vi "Zwangsbedingungen-04-02-17.vi"(4 "AnzahlHorst":i32, 5 "AnzahlHorst/Modul":i32[](array[numeric]), 6 "AnzahlLH":i32, 7 "AnzahlDIOs/Modul":i32[](array[numeric]), 8 "AnzahlDIOs":i32, 9 "Zwangsbedingungen":dbl[][](array[numeric]), 10 "Methodennummer":i32(ring) items=["0"]) -> (1 "Methodennummer":i32(ring) items=["0"])   [LabVIEW 2010]
uses:
  GVMWHorst.vi
  GVHK1Hz.vi
  gvbooleschRT.vi
  GVZeitenZyklen.vi
  GVVentilposition.vi
  GVMetavariablen.vi
  GVZwangs.vi
  GVZwangsMPVPos.vi
  GVZwangsMPV.vi
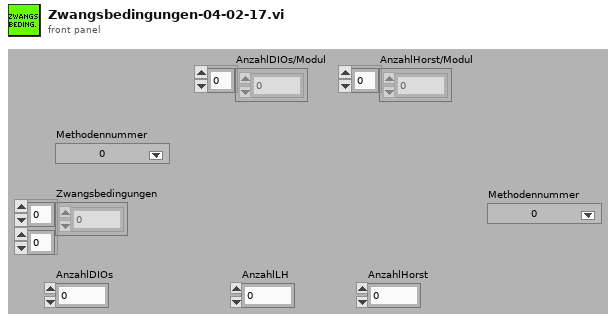
[diagram p1: front panel]
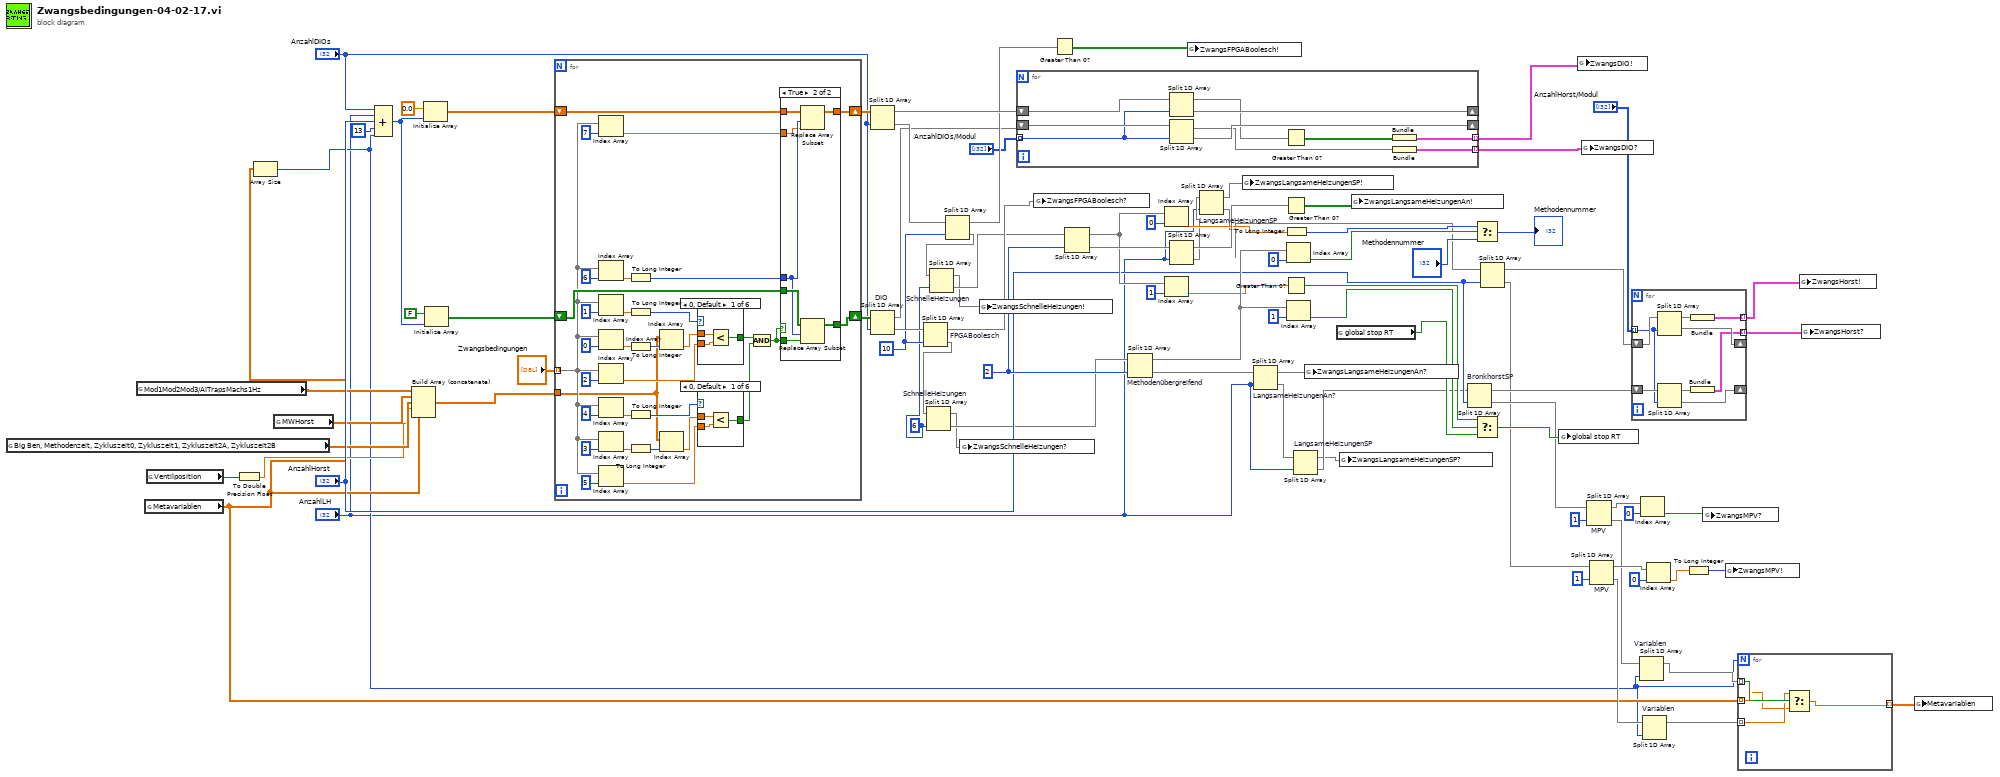
[diagram p0: block diagram]
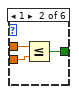
[diagram p2: hidden frame]
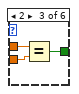
[diagram p3: hidden frame]
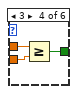
[diagram p4: hidden frame]
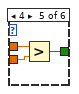
[diagram p5: hidden frame]
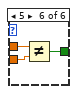
[diagram p6: hidden frame]
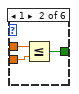
[diagram p8: hidden frame]
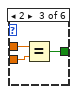
[diagram p9: hidden frame]
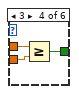
[diagram p10: hidden frame]
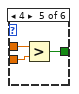
[diagram p11: hidden frame]
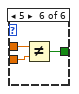
[diagram p12: hidden frame]
diagram:
  w10 = 6 ("index")
  w74 = 2 ("Index")
  w81 = 10 ("Index")
  n1 = global read "GVZeitenZyklen.vi" "Big Ben, Methodenzeit, Zykluszeit0, Zykluszeit1, Zykluszeit2A, Zykluszeit2B"() -> (w35:dbl[])
  n2 = global read "GVHK1Hz.vi" "Mod1Mod2Mod3/AITrapsMachs1Hz"() -> (w38:dbl[])
  n3 = global read "GVMetavariablen.vi" "Metavariablen"() -> (w16:dbl[])
  n4 = global read "GVVentilposition.vi" "Ventilposition"() -> (w34:i32)
  n5 = To Double Precision Float(number=w34) -> (double precision float=w33:dbl)
  n6 = Array Size(array=w16) -> (size(s)=w15:i32)
  n7 = global read "GVMWHorst.vi" "MWHorst"() -> (w47:dbl[])
  n8 = Compound Arithmetic op=ADD("AnzahlDIOs", "AnzahlLH", "AnzahlHorst", 13 ("Wert"), w15) -> (w63:i32)
  n9 = Build Array (concatenate)(w38, w47, w35, w33, w16) -> (w87:dbl[])
  n10 = Initialize Array(0.0, w63) -> (w60:dbl[])
  n11 = Initialize Array(FALSE, w63) -> (w59:bool[])
  n12 = for {
    tunnel: w87 -> [w94]
    tunnel: "Zwangsbedingungen" -> [w98] mode=indexing
    shift-right: [w102] -> w86
    shift-left: w59 -> [w107]
    shift-right: [w103] -> w83
    shift-left: w60 -> [w106]
    n13 = Index Array(array=w98, index=7 ("Index")) -> (element=w104:dbl)
    n14 = Index Array(array=w98, index=6 ("Index")) -> (element=w109:dbl)
    n15 = Index Array(array=w98, index=1 ("Index")) -> (element=w116:dbl)
    n16 = Index Array(array=w98, index=0 ("Index")) -> (element=w118:dbl)
    n17 = Index Array(array=w98, index=2 ("Index")) -> (element=w112:dbl)
    n18 = Index Array(array=w98, index=4 ("Index")) -> (element=w92:dbl)
    n19 = Index Array(array=w98, index=3 ("Index")) -> (element=w93:dbl)
    n20 = Index Array(array=w98, index=5 ("Index")) -> (element=w91:dbl)
    n21 = To Long Integer(number=w109) -> (32bit integer=w105:i32)
    n22 = To Long Integer(number=w116) -> (32bit integer=w115:i32)
    n23 = To Long Integer(number=w118) -> (32bit integer=w111:i32)
    n24 = To Long Integer(number=w92) -> (32bit integer=w97:i32)
    n25 = To Long Integer(number=w93) -> (32bit integer=w95:i32)
    n26 = Index Array(array=w94, index=w111) -> (element=w114:dbl)
    n27 = Index Array(array=w94, index=w95) -> (element=w96:dbl)
    n28 = case shown="0, Default" w115 {
      tunnel: w114 -> [w149 w151 w155 w158 w161 w164]
      tunnel: w112 -> [w148 w152 w154 w157 w160 w163]
      tunnel: [w147 w150 w153 w156 w159 w162] -> w89
      frame 0, Default {
        n29 = Less?(x=w149, y=w148) -> (x < y?=w147:bool)
      }
      frame 1 {
        n30 = Less Or Equal?(x=w151, y=w152) -> (x <= y?=w150:bool)
      }
      frame 2 {
        n31 = Equal?(x=w155, y=w154) -> (x = y?=w153:bool)
      }
      frame 3 {
        n32 = Greater Or Equal?(x=w158, y=w157) -> (x >= y?=w156:bool)
      }
      frame 4 {
        n33 = Greater?(x=w161, y=w160) -> (0:w159:bool)
      }
      frame 5 {
        n34 = Not Equal?(x=w164, y=w163) -> (x != y?=w162:bool)
      }
    }
    n35 = case shown="0, Default" w97 {
      tunnel: w96 -> [w122 w124 w128 w131 w134 w137]
      tunnel: w91 -> [w121 w125 w127 w130 w133 w136]
      tunnel: [w120 w123 w126 w129 w132 w135] -> w90
      frame 0, Default {
        n36 = Less?(x=w122, y=w121) -> (x < y?=w120:bool)
      }
      frame 1 {
        n37 = Less Or Equal?(x=w124, y=w125) -> (x <= y?=w123:bool)
      }
      frame 2 {
        n38 = Equal?(x=w128, y=w127) -> (x = y?=w126:bool)
      }
      frame 3 {
        n39 = Greater Or Equal?(x=w131, y=w130) -> (x >= y?=w129:bool)
      }
      frame 4 {
        n40 = Greater?(x=w134, y=w133) -> (0:w132:bool)
      }
      frame 5 {
        n41 = Not Equal?(x=w137, y=w136) -> (x != y?=w135:bool)
      }
    }
    n42 = And(x=w89, y=w90) -> (x .and. y?=w88:bool)
    n43 = case shown="True" w88 {
      tunnel: w107 -> [w139 w146]
      tunnel: w106 -> [w138 w145]
      tunnel: w105 -> [_ w144]
      tunnel: w88 -> [_ w143]
      tunnel: w104 -> [_ w142]
      tunnel: [w138 w141] -> w103
      tunnel: [w139 w140] -> w102
      frame False {
      }
      frame True {
        n44 = Replace Array Subset(array=w145, new element=w142, index=w144) -> (w141:dbl[])
        n45 = Replace Array Subset(array=w146, new element=w143, index=w144) -> (w140:bool[])
      }
    }
  }
  n46 = Split 1D Array ("DIO")(array=w83, index="AnzahlDIOs") -> (first subarray=w82:dbl[], second subarray=w80:dbl[])
  n47 = Split 1D Array "DIO"(array=w86, index="AnzahlDIOs") -> (first subarray=w69:bool[], second subarray=w85:bool[])
  n48 = Split 1D Array "FPGABoolesch"(array=w85, index=w81) -> (first subarray=w46:bool[], second subarray=w14:bool[])
  n49 = Split 1D Array "SchnelleHeizungen"(array=w14, index=w10) -> (first subarray=w12:bool[], second subarray=w13:bool[])
  n50 = Split 1D Array(array=w80, index=w81) -> (first subarray=w79:dbl[], second subarray=w11:dbl[])
  n51 = Split 1D Array "SchnelleHeizungen"(array=w11, index=w10) -> (first subarray=w8:dbl[], second subarray=w9:dbl[])
  n52 = global write "GVZwangs.vi" "ZwangsSchnelleHeizungen?"(w12) -> ()
  n53 = global write "GVZwangs.vi" "ZwangsSchnelleHeizungen!"(w8) -> ()
  n54 = for {
    tunnel: [w167] -> w41 mode=indexing
    tunnel: "AnzahlDIOs/Modul" -> [w169] mode=indexing
    tunnel: [w165] -> w42 mode=indexing
    shift-right: [w173] -> _
    shift-left: w69 -> [w174]
    shift-right: [w171] -> _
    shift-left: w82 -> [w172]
    n55 = Split 1D Array(array=w172, index=w169) -> (first subarray=w170:dbl[], second subarray=w171:dbl[])
    n56 = Split 1D Array(array=w174, index=w169) -> (first subarray=w168:bool[], second subarray=w173:bool[])
    n57 = Greater Than 0?(x=w170) -> (x > 0?=w166:bool[])
    n58 = Bundle(w166) -> (w165:cluster{bool[]})  [unwired: 1 in]
    n59 = Bundle(w168) -> (w167:cluster{bool[]})  [unwired: 1 in]
  }
  n60 = global write "GVZwangs.vi" "ZwangsFPGABoolesch?"(w46) -> ()
  n61 = Greater Than 0?(x=w79) -> (x > 0?=w45:bool[])
  n62 = Split 1D Array(array=w9, index=w74) -> (first subarray=w70:dbl[], second subarray=w75:dbl[])
  n63 = Split 1D Array "Methodenübergreifend"(array=w13, index=w74) -> (first subarray=w72:bool[], second subarray=w76:bool[])
  n64 = Index Array(array=w70, index=0 ("Index")) -> (element=w52:dbl)
  n65 = Index Array(array=w70, index=1 ("Index")) -> (element=w56:dbl)
  n66 = Split 1D Array(array=w75, index="AnzahlLH") -> (first subarray=w77:dbl[], second subarray=w4:dbl[])
  n67 = global write "GVZwangs.vi" "ZwangsFPGABoolesch!"(w45) -> ()
  n68 = Split 1D Array "LangsameHeizungenSP"(array=w4, index="AnzahlLH") -> (first subarray=w1:dbl[], second subarray=w2:dbl[])
  n69 = global write "GVZwangs.vi" "ZwangsLangsameHeizungenSP!"(w1) -> ()
  n70 = Split 1D Array "LangsameHeizungenAn?"(array=w76, index="AnzahlLH") -> (first subarray=w44:bool[], second subarray=w7:bool[])
  n71 = Greater Than 0?(x=w77) -> (x > 0?=w43:bool[])
  n72 = To Long Integer(number=w52) -> (32bit integer=w50:i32)
  n73 = Greater Than 0?(x=w56) -> (x > 0?=w54:bool)
  n74 = Index Array(array=w72, index=0 ("Index")) -> (element=w51:bool)
  n75 = Index Array(array=w72, index=1 ("Index")) -> (element=w55:bool)
  n76 = Split 1D Array "LangsameHeizungenSP"(array=w7, index="AnzahlLH") -> (first subarray=w5:bool[], second subarray=w6:bool[])
  n77 = global write "GVZwangs.vi" "ZwangsLangsameHeizungenAn?"(w44) -> ()
  n78 = global read "gvbooleschRT.vi" "global stop RT"() -> (w37:bool)
  n79 = global write "GVZwangs.vi" "ZwangsLangsameHeizungenSP?"(w5) -> ()
  n80 = global write "GVZwangs.vi" "ZwangsLangsameHeizungenAn!"(w43) -> ()
  n81 = Split 1D Array "BronkhorstSP"(array=w6, index="AnzahlHorst") -> (first subarray=w84:bool[], second subarray=w32:bool[])
  n82 = Select(t=w50, s=w51, f="Methodennummer") -> (s? t:f=→"Methodennummer":i32)
  n83 = Select(t=w54, s=w55, f=w37) -> (s? t:f=w36:bool)
  n84 = Split 1D Array(array=w2, index="AnzahlHorst") -> (first subarray=w78:dbl[], second subarray=w29:dbl[])
  n85 = global write "gvbooleschRT.vi" "global stop RT"(w36) -> ()
  n86 = global write "GVZwangs.vi" "ZwangsDIO!"(w42) -> ()
  n87 = global write "GVZwangs.vi" "ZwangsDIO?"(w41) -> ()
  n88 = Split 1D Array "MPV"(array=w32, index=1 ("Index")) -> (first subarray=w28:bool[], second subarray=w21:bool[])
  n89 = Split 1D Array "MPV"(array=w29, index=1 ("Index")) -> (first subarray=w24:dbl[], second subarray=w20:dbl[])
  n90 = for {
    tunnel: "AnzahlHorst/Modul" -> [w180] mode=indexing
    shift-right: [w182] -> _
    shift-left: w84 -> [w183]
    tunnel: [w177] -> w39 mode=indexing
    shift-right: [w179] -> _
    shift-left: w78 -> [w181]
    tunnel: [w175] -> w40 mode=indexing
    n91 = Split 1D Array(array=w181, index=w180) -> (first subarray=w176:dbl[], second subarray=w179:dbl[])
    n92 = Split 1D Array(array=w183, index=w180) -> (first subarray=w178:bool[], second subarray=w182:bool[])
    n93 = Bundle(w176) -> (w175:cluster{dbl[]})  [unwired: 1 in]
    n94 = Bundle(w178) -> (w177:cluster{bool[]})  [unwired: 1 in]
  }
  n95 = Split 1D Array "Variablen"(array=w21, index=w15) -> (first subarray=w19:bool[])  [unwired: 1 out]
  n96 = Index Array(array=w28, index=0 ("Index")) -> (element=w26:bool)
  n97 = Split 1D Array "Variablen"(array=w20, index=w15) -> (first subarray=w18:dbl[])  [unwired: 1 out]
  n98 = Index Array(array=w24, index=0 ("Index")) -> (element=w23:dbl)
  n99 = To Long Integer(number=w23) -> (32bit integer=w22:i32)
  n100 = global write "GVZwangsMPV.vi" "ZwangsMPV?"(w26) -> ()
  n101 = global write "GVZwangsMPVPos.vi" "ZwangsMPV!"(w22) -> ()
  n102 = for {
    N: w15 -> [_]
    tunnel: w19 -> [w187] mode=indexing
    tunnel: w18 -> [w186] mode=indexing
    tunnel: w16 -> [w185] mode=indexing
    tunnel: [w184] -> w17 mode=indexing
    n103 = Select(t=w186, s=w187, f=w185) -> (s? t:f=w184:dbl)
  }
  n104 = global write "GVZwangs.vi" "ZwangsHorst!"(w40) -> ()
  n105 = global write "GVZwangs.vi" "ZwangsHorst?"(w39) -> ()
  n106 = global write "GVMetavariablen.vi" "Metavariablen"(w17) -> ()
